vi "Convert Detection Ball to AI Ball.vi"(7 "Lado":enum16{"Esquerdo", "Direito"}(ring) caption="Enum", 10 "SSL Vision":bool, 11 "Input":T2[](array[typedef])) -> (3 "Output":T1[](array[typedef]))   [LabVIEW 2018]
uses:
  SSL Detection Ball.ctl
  <vilib>/Analysis/Matrix/Datatypes/RealMatrix.ctl
  AI Ball.ctl
  <vilib>/Analysis/Matrix/NI_Matrix.lvlib
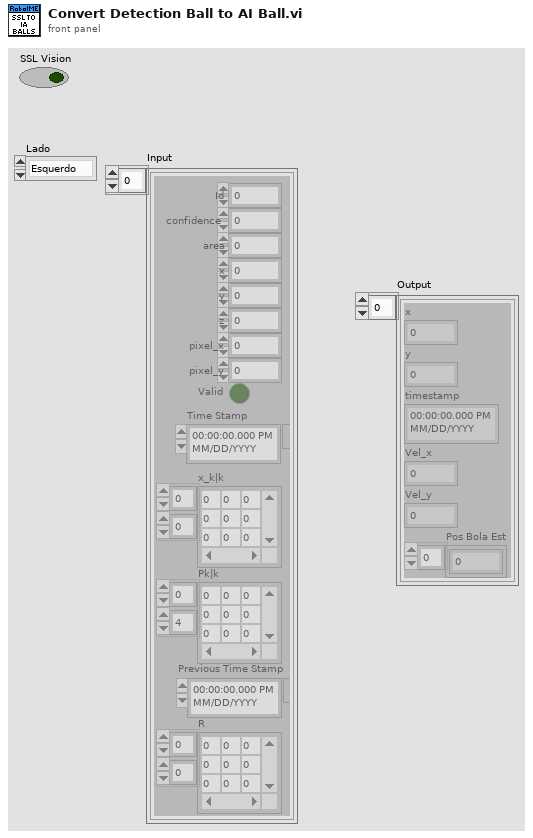
[diagram p1: front panel]
types:
  T1 = typedef "AI Ball.ctl" = cluster{"x":dbl, "y":dbl, "timestamp":timestamp, "Vel_x":dbl, "Vel_y":dbl, "Pos Bola Est":dbl[]}
  T2 = typedef "SSL Detection Ball.ctl" = cluster{"x":sgl, "area":u32, "confidence":sgl, "y":sgl, "z":sgl, "pixel_x":sgl, "pixel_y":sgl, "Valid":bool, "Time Stamp":timestamp, "x_k|k":T3, "Pk|k":T3, "Id":u32, "Previous Time Stamp":timestamp, "R":T3}
  T3 = typedef "NI_Matrix.lvlib/RealMatrix.ctl" = dbl[][]
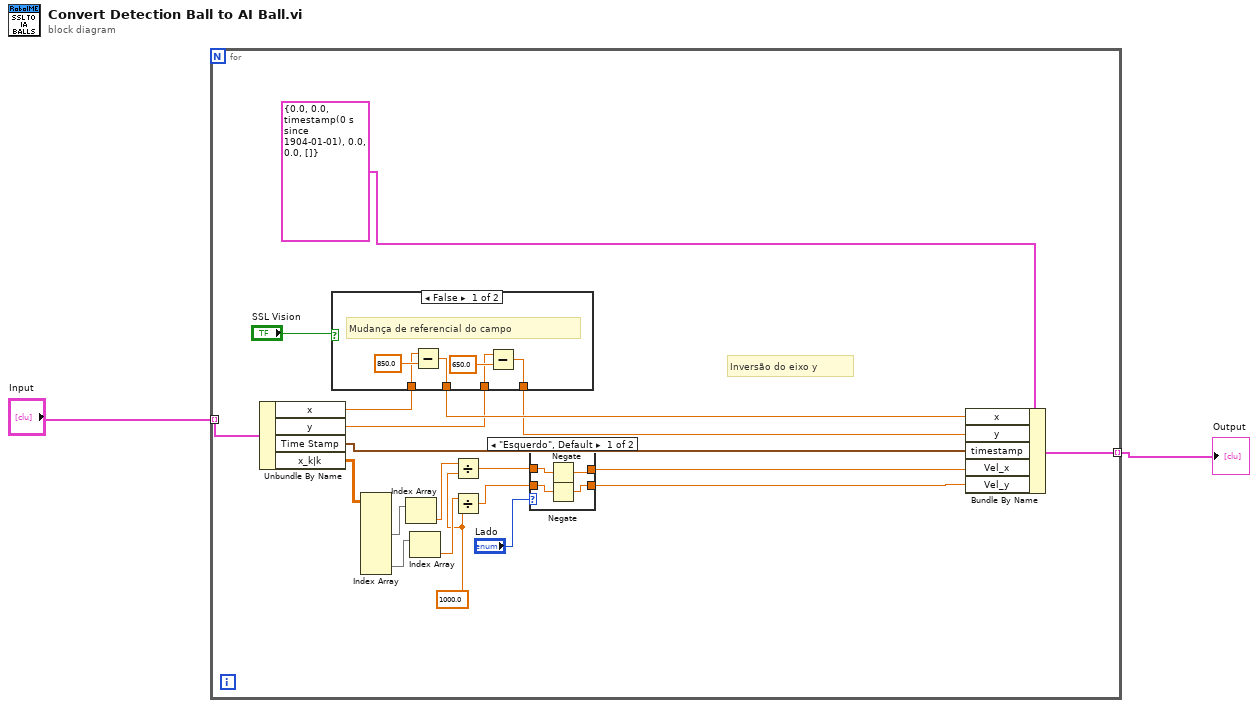
[diagram p0: block diagram]
diagram:
  n1 = for {
    tunnel: "Input" -> [w21] mode=indexing
    tunnel: [w20] -> w1 mode=indexing
    w13 = 1000.0
    # "Inversão do eixo y"
    n2 = Unbundle By Name(w21) -> ("x"=w7:sgl, "y"=w5:sgl, "Time Stamp"=w19:timestamp, "x_k|k"=w18:T3)
    n3 = case shown="False" "SSL Vision" {
      tunnel: w7 -> [w27 w30]
      tunnel: [w26 w30] -> w6
      tunnel: w5 -> [w24 w29]
      tunnel: [w23 w29] -> w4
      frame False {
        # "Mudança de referencial do campo"
        n4 = Subtract(x=w27, y=850.0) -> (x-y=w26:dbl)
        n5 = Subtract(x=w24, y=650.0) -> (x-y=w23:dbl)
      }
      frame True {
      }
    }
    n6 = Index Array(array=w18) -> (element #2=w17:dbl[], element #4=w16:dbl[])  [unwired: 8 in, 2 out]
    n7 = Index Array(array=w17) -> (element=w15:dbl)  [unwired: 1 in]
    n8 = Index Array(array=w16) -> (element=w14:dbl)  [unwired: 1 in]
    n9 = Divide(x=w15, y=w13) -> (x/y=w11:dbl)
    n10 = Divide(x=w14, y=w13) -> (x/y=w8:dbl)
    n11 = case shown="\"Esquerdo\", Default" "Lado" {
      tunnel: [w34 w36] -> w10
      tunnel: w11 -> [w33 w36]
      tunnel: [w31 w35] -> w9
      tunnel: w8 -> [w32 w35]
      frame "Esquerdo", Default {
        n12 = Negate(x=w33) -> (-x=w34:dbl)
        n13 = Negate(x=w32) -> (-x=w31:dbl)
      }
      frame "Direito" {
      }
    }
    n14 = Bundle By Name(cluster=T1 {"x"=0.0, "y"=0.0, "timestamp"=timestamp(0 s since 1904-01-01), "Vel_x"=0.0, "Vel_y"=0.0, "Pos Bola Est"=[]} ("Ball"), "x"=w6, "y"=w4, "timestamp"=w19, "Vel_x"=w10, "Vel_y"=w9) -> (w20:T1)
  }
  "Output" <- w1
